vi "Initialize Configuration Resource.vi"(8 "error in (no error)":errorcluster, 11 "IConfiguration in":refnum<class "IConfiguration.lvclass">) -> (0 "error out":errorcluster, 3 "IConfiguration out":refnum<class "IConfiguration.lvclass">)   [LabVIEW 2017, in "Configuration.lvlib" / "IConfiguration.lvclass"]
uses:
  IConfiguration.lvclass
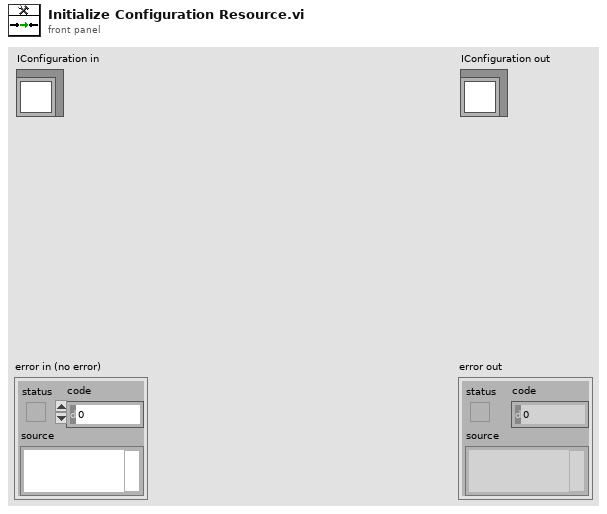
[diagram p1: front panel]
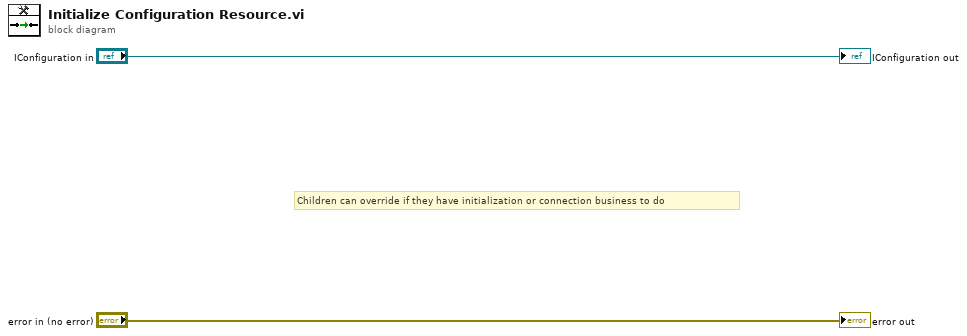
[diagram p0: block diagram]
diagram:
  # "Children can override if they have initialization or connection business to do"
  "error out" <- "error in (no error)"
  "IConfiguration out" <- "IConfiguration in"
